vi "Solve1.vi"(8 "Error In":errorcluster, 11 "object in":refnum<class "2022_3.lvclass">) -> (0 "Error Out":errorcluster, 2 "Result":u64, 3 "object out":refnum<class "2022_3.lvclass">)   [LabVIEW 2020, in "2022_3.lvclass"]
uses:
  2022_3.lvclass
  2022_3.lvclass/2022_3.ctl
  f60bf04f-f187-4e0f-8b1d-92790ebf2850.vi
  d897a993-7c79-4cdb-aa70-7bfd256bd790.vi
  e5abeff6-d601-4f1e-a2ca-bc693e0ea41f.vi
  f60bf04f-f187-4e0f-8b1d-92790ebf2850.vi/be6f088c-3e4b-4523-ad48-2cdc85bad38a.vi
  f60bf04f-f187-4e0f-8b1d-92790ebf2850.vi/f202eadf-433e-4cdb-b986-b2351ce8d73c.vi
  f60bf04f-f187-4e0f-8b1d-92790ebf2850.vi/094751bc-bcf2-4346-afae-53942128b536.vi
  f60bf04f-f187-4e0f-8b1d-92790ebf2850.vi/06ee343e-764f-4086-89d5-f578778d243c.vi
panel:
  out "Letter":string
  out "elements":u8[](array[numeric])
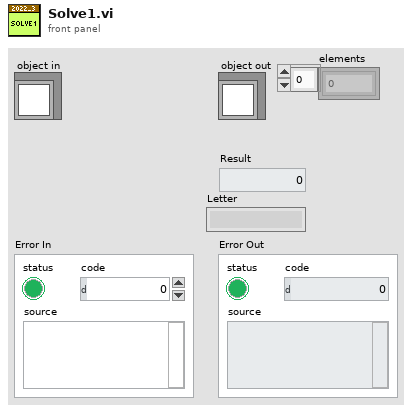
[diagram p1: front panel]
types:
  T1 = cluster{"Compartment1":u8[], "Compartment2":u8[]}[]
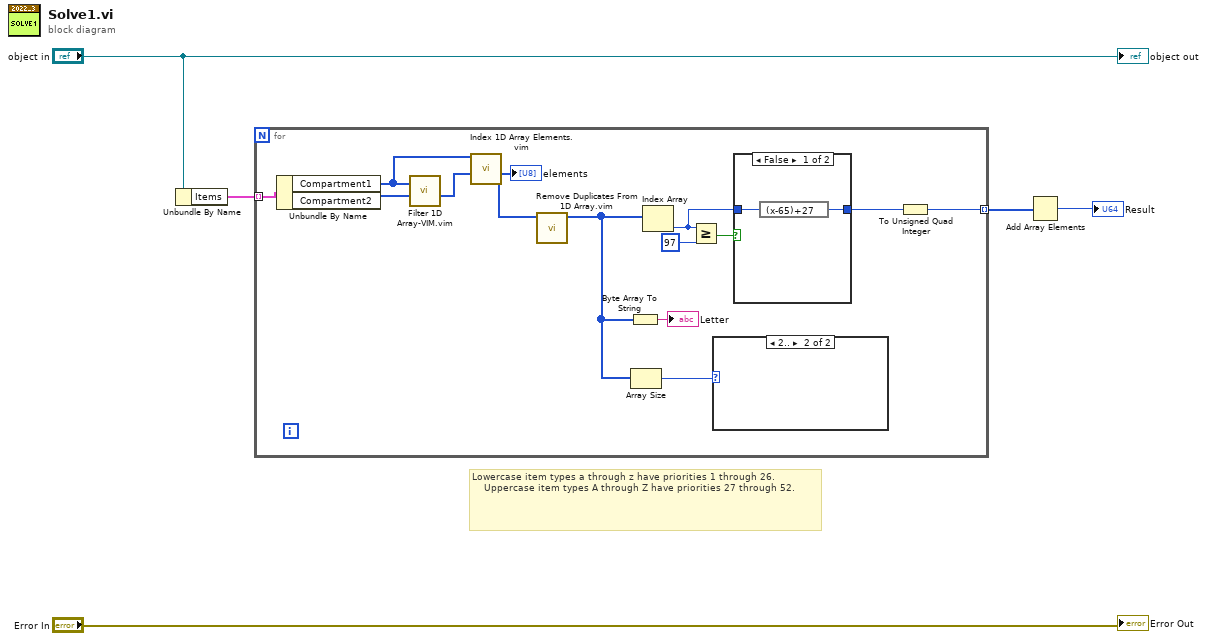
[diagram p0: block diagram]
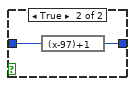
[diagram p2: hidden frame]
diagram:
  # "Lowercase item types a through z have priorities 1 through 26.\n    Uppercase item types A through Z have priorities 27 through 52."
  n1 = Unbundle By Name("object in") -> ("Items"=w3:T1)
  n2 = for {
    tunnel: w3 -> [w18] mode=indexing
    tunnel: [w8] -> w2 mode=indexing
    n3 = Unbundle By Name(w18) -> ("Compartment1"=w16:u8[], "Compartment2"=w17:u8[])
    n4 = call "Filter 1D Array-VIM.vim"("Item(s) to Filter"=w17, "Array"=w16) -> ("Filtered Item Indices"=w15:i32[])  [unwired: 5 in, 1 out]
    n5 = call "Index 1D Array Elements.vim"("indices"=w15, "array"=w16) -> ("elements"=w14:u8[])  [unwired: 9 in]
    "elements" <- w14
    n6 = call "Remove Duplicates From 1D Array.vim"("array"=w14) -> ("array with duplicates removed"=w7:u8[])  [unwired: 10 in]
    n7 = Byte Array To String(unsigned byte array=w7) -> (string=→"Letter":string)
    n8 = Array Size(array=w7) -> (size(s)=w13:i32)
    n9 = Index Array(array=w7) -> (element=w10:u8)  [unwired: 1 in]
    n10 = Greater Or Equal?(x=w10, y=u8 97) -> (x >= y?=w11:bool)
    n11 = case shown="2.." w13 {
      frame 0, Default {
      }
      frame 2.. {
      }
    }
    n12 = case shown="False" w11 {
      tunnel: w10 -> [w20 w22]
      tunnel: [w19 w21] -> w9
      frame False {
        n13 = expression code="(x-65)+27"(w20) -> (w19:u8)
      }
      frame True {
        n14 = expression code="(x-97)+1"(w22) -> (w21:u8)
      }
    }
    n15 = To Unsigned Quad Integer(1:w9) -> (0:w8:u64)
  }
  n16 = Add Array Elements(numeric array=w2) -> (sum=→"Result":u64)
  "Error Out" <- "Error In"
  "object out" <- "object in"
